vi "DAQ DI_EStop.vi"(8 "error in":errorcluster, 11 "Alias":string) -> (0 "error out":errorcluster, 3 "DI out":bool)   [LabVIEW 2021]
uses:
  DAQ_Data.ctl
  Measure Type.ctl
  <vilib>/DAQmx/read.llb/DAQmx Read (Digital Bool 1Line 1Point).vi
  <vilib>/DAQmx/create/channels.llb/DAQmx Create Channel (DI-Digital Input).vi
  <vilib>/DAQmx/miscellaneous.llb/DAQmx Fill In Error Info.vi
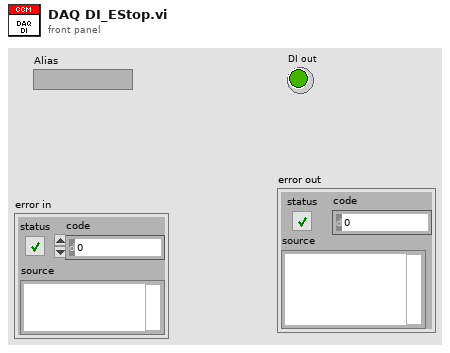
[diagram p1: front panel]
types:
  T1 = typedef "Measure Type.ctl" = enum16{"Analog In", "Analog Out", "Digital In", "Digital Out", "Switch", "NI DMM"}
  T2 = typedef "DAQ_Data.ctl" = cluster{"Alias":string, "DAQ Ch":string}
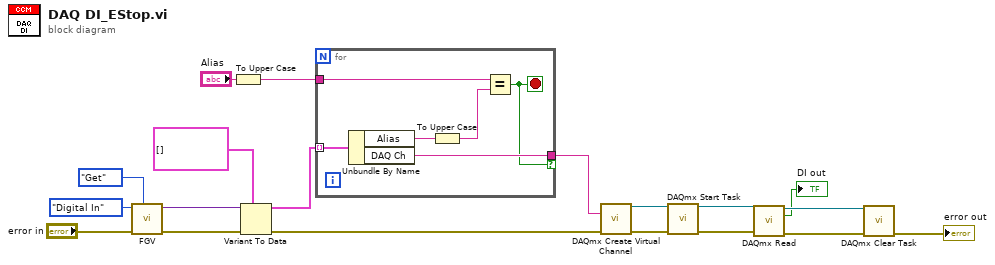
[diagram p0: block diagram]
diagram:
  n1 = call "FGV.vi"("Method (Get)"=enum16{"Get", "Set"}."Get", "error in"="error in", "Name"=Measure_Type."Digital In") -> ("error out"=w13:errorcluster, "Data out"=w12:variant)  [unwired: 7 in]
  n2 = To Upper Case(1:"Alias") -> (0:w2:string)
  n3 = Variant To Data(error in=w13, type=T2[] [], Variant=w12) -> (data=w4:T2[], error out=w9:errorcluster)
  n4 = for {
    tunnel: w4 -> [w25] mode=indexing
    tunnel: [w24] -> w1 if=w21
    tunnel: w2 -> [w23]
    stop <- w21 stop-if-true
    n5 = Unbundle By Name(w25) -> ("Alias"=w22:string, "DAQ Ch"=w24:string)
    n6 = To Upper Case(1:w22) -> (0:w20:string)
    n7 = Equal?(x=w23, y=w20) -> (x = y?=w21:bool)
  }
  n8 = call-poly <vilib>:"DAQmx Create Virtual Channel.vi"("lines"=w1, "error in"=w9) -> ("task out"=w17:refnum<k21>, "error out"=w18:errorcluster)  [unwired: 12 in]
  n9 = call <vilib>:"DAQmx Start Task.vi"("task/channels in"=w17, "error in"=w18) -> ("task out"=w6:refnum<k21>, "error out"=w5:errorcluster)  [unwired: 12 in]
  n10 = call-poly <vilib>:"DAQmx Read.vi"("task/channels in"=w6, "error in"=w5) -> ("task out"=w16:refnum<k21>, "data"=→"DI out":bool, "error out"=w15:errorcluster)  [unwired: 11 in]
  n11 = call <vilib>:"DAQmx Clear Task.vi"("task in"=w16, "error in"=w15) -> ("error out"=→"error out":errorcluster)  [unwired: 13 in]
